vi "Update display.vi"(8 "Error In":errorcluster, 10 "Display states":T1, 11 "Cluster":T2) -> (0 "Error Out":errorcluster)   [LabVIEW 2020, in "Test Framework.lvclass"]
uses:
  Test Framework.lvclass
  Controls/Control references.ctl
  Controls/Display states.ctl
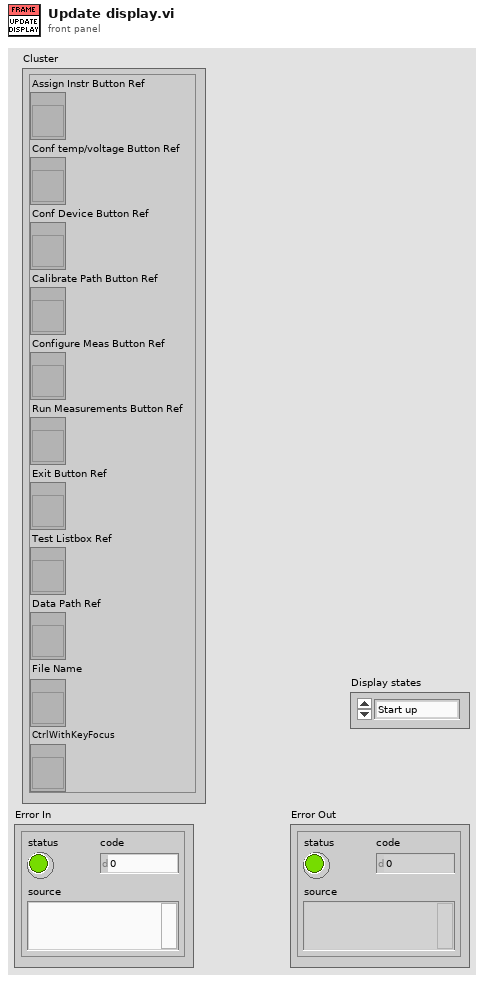
[diagram p1: front panel]
types:
  T1 = typedef "Test Framework.lvclass/Display states.ctl" = enum16{"Start up", "Measurements Running"}
  T2 = typedef "Test Framework.lvclass/Control references.ctl" = cluster{"Assign Instr Button Ref":refnum<vi>, "Conf temp/voltage Button Ref":refnum<vi>, "Conf Device Button Ref":refnum<vi>, "Calibrate Path Button Ref":refnum<vi>, "Configure Meas Button Ref":refnum<vi>, "Run Measurements Button Ref":refnum<vi>, "Exit Button Ref":refnum<vi>, "Test Listbox Ref":refnum<vi>, "Data Path Ref":refnum<vi>, "File Name":refnum<vi>, "CtrlWithKeyFocus":refnum<vi>}
  T3 = enum8{"Enabled", "Disabled", "Disabled and Grayed Out"}
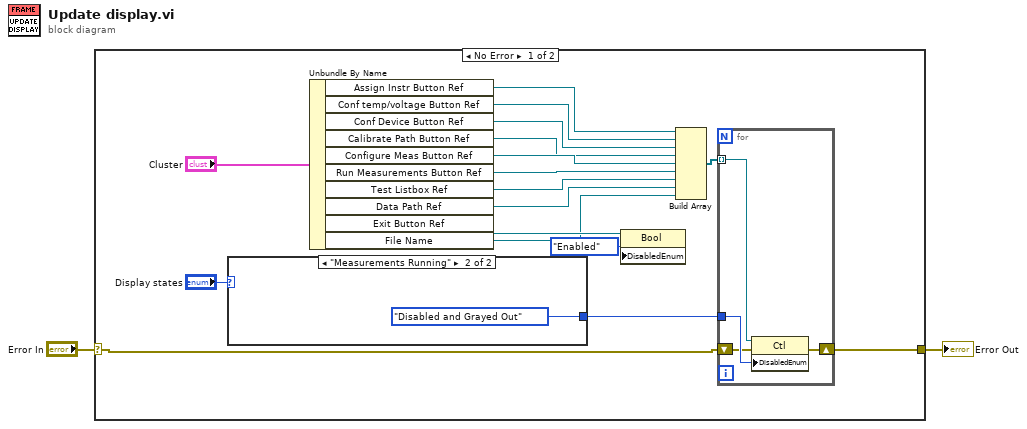
[diagram p0: block diagram]
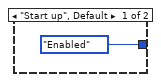
[diagram p2: hidden frame]
diagram:
  n1 = case shown="No Error" "Error In" {
    selector: "Error In" -> [w4 w26]
    tunnel: [w7 w26] -> w2
    frame No Error {
      n2 = case shown="\"Measurements Running\"" "Display states" {
        tunnel: [T3."Enabled" ("Disabled") T3."Disabled and Grayed Out" ("Disabled")] -> w8
        frame "Start up", Default {
        }
        frame "Measurements Running" {
        }
      }
      n3 = Unbundle By Name("Cluster") -> ("Assign Instr Button Ref"=w11:refnum<vi>, "Conf temp/voltage Button Ref"=w12:refnum<vi>, "Conf Device Button Ref"=w13:refnum<vi>, "Calibrate Path Button Ref"=w14:refnum<vi>, "Configure Meas Button Ref"=w15:refnum<vi>, "Run Measurements Button Ref"=w16:refnum<vi>, "Test Listbox Ref"=w17:refnum<vi>, "Data Path Ref"=w18:refnum<vi>, "Exit Button Ref"=w6:refnum<vi>, "File Name"=w3:refnum<vi>)
      n4 = property class="Bool"(reference=w6, "DisabledEnum"=T3."Enabled" ("Disabled")) -> ()  [unwired: 1 in, 2 out]
      n5 = Build Array(w11, w12, w13, w14, w15, w16, w17, w18, w3) -> (w10:refnum<vi>[])
      n6 = for {
        tunnel: w10 -> [w25] mode=indexing
        tunnel: w8 -> [w24]
        shift-right: [w22] -> w7
        shift-left: w4 -> [w23]
        n7 = property class="Ctl"(reference=w25, error in=w23, "DisabledEnum"=w24) -> (error out=w22:errorcluster)  [unwired: 1 out]
      }
    }
    frame Error {
    }
  }
  "Error Out" <- w2
